vi "GlobalVar.vi"() -> ()   [LabVIEW 2017]
panel:
  in  "r_wheel":dbl
  in  "r_car":dbl
  out "servo 3":u8
  out "servo 2":u8
  out "servo 1":u8
  in  "MOTOR_POW":i8
  in  "R_MOTOR_POS":i32
  in  "L_MOTOR_POS":i32
  # "= 269.54 mm"
  # "= 101.5 mm"
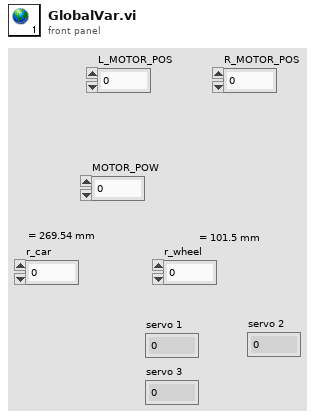
[diagram p1: front panel]
diagram:
